vi "File Page - Get Stop Trigger.vi"(7 "File Ctl Refs":T1, 8 "error in (no error)":errorcluster, 11 "Item Ref in":T11 format="%.0x") -> (0 "error out":errorcluster, 3 "Item Ref out":T11 format="%.0x")   [LabVIEW 2015, in "Waveform Data Logger System Explorer.lvlib"]
uses:
  Waveform Data Logger System Explorer.lvlib
  <vilib>/NI Veristand/Custom Device API/Custom Device Item Ref.ctl
  Types/File Ctl Refs.ctl
  Types/File - Spec Ctl Refs.ctl
  Types/File - Wfm Ctl Refs.ctl
  Types/File - Settings Ctl Refs.ctl
  Classes/Log File Specifications/Log File Specification/File Conflict Operation.ctl
  Types/File - Start Trig Ctl Refs.ctl
  Shared/Types/Start Trigger.ctl
  Shared/Types/Default Trigger.ctl
  Shared/Types/Digital Trigger.ctl
  Shared/Types/Analog Trigger.ctl
  Shared/Types/In Range Trigger.ctl
  Shared/Types/Value Change Trigger.ctl
  Shared/Types/Boolean Trigger.ctl
  Types/Single Node Browser Data.ctl
  <vilib>/NI Veristand/UI Controls/Single Node Browser/Single Node Browser Ref.ctl
  NationalInstruments.VeriStand.SystemStorageUI
  <vilib>/NI Veristand/UI Controls/Single Node Browser/Callback Type.ctl
  <vilib>/NI Veristand/UI Controls/Single Node Browser/Net Event Data.ctl
  <vilib>/NI Veristand/UI Controls/Single Node Browser/Net Event.ctl
  Types/File - Stop Trig Ctl Refs.ctl
  Shared/Types/Stop Trigger.ctl
  Types/File - Advanced Ctl Refs.ctl
  Types/Log Timestamps.ctl
  Shared/Types/Trigger Direction.ctl
  Shared/Globals/Property Strings.vi
  <vilib>/NI Veristand/Custom Device API/Get Item Property (U16).vi
  <vilib>/NI Veristand/Custom Device API/Get Item Property (Double).vi
  Shared/Waveform Data Logger Shared.lvlib
  <vilib>/NI Veristand/Custom Device API/Custom Device API.lvlib
  Classes/Log File Specifications/Log File Specification/Log File Specification.lvclass
  <vilib>/NI Veristand/UI Controls/Single Node Browser/NI_VS UI Single Node Browser.lvlib
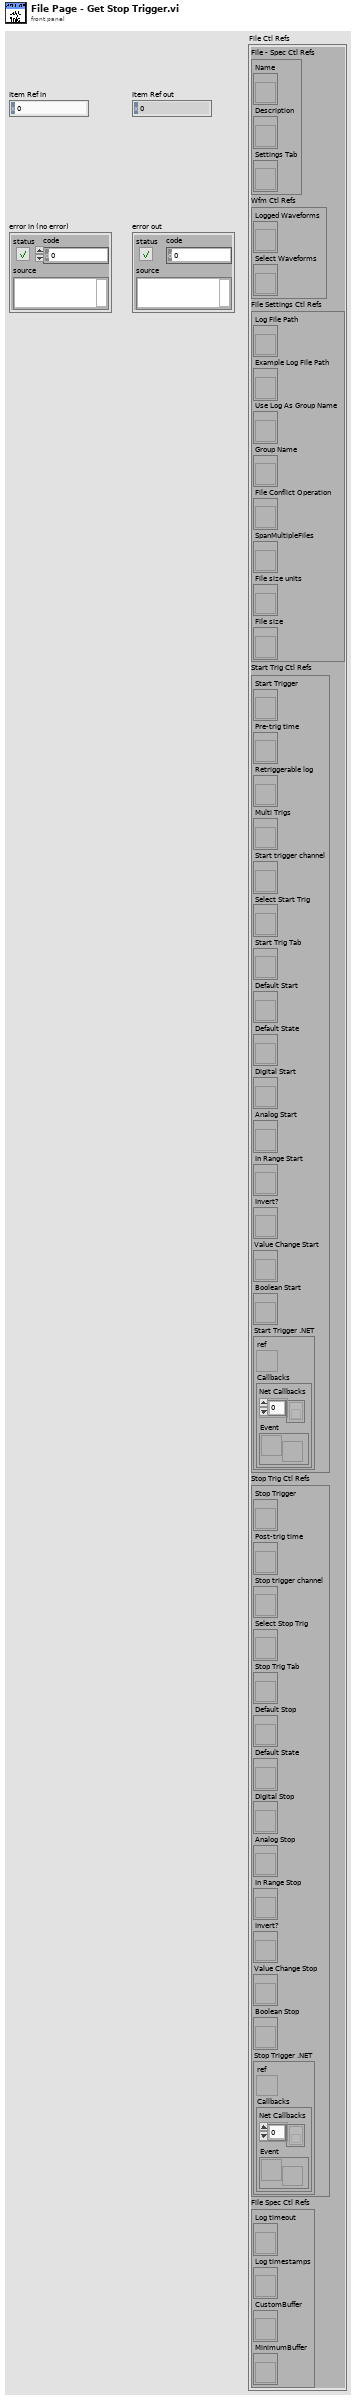
[diagram p1: front panel]
types:
  T1 = typedef "Waveform Data Logger System Explorer.lvlib/File Ctl Refs.ctl" = cluster{"File Spec Ctl Refs":T2, "Wfm Ctl Refs":T3, "File Settings Ctl Refs":T4, "Start Trig Ctl Refs":T5, "Stop Trig Ctl Refs":T9, "File Spec Ctl Refs":T10}
  T2 = typedef "Waveform Data Logger System Explorer.lvlib/File - Spec Ctl Refs.ctl" = cluster{"Name":refnum<vi>, "Description":refnum<vi>, "Settings Tab":refnum<vi>}
  T3 = typedef "Waveform Data Logger System Explorer.lvlib/File - Wfm Ctl Refs.ctl" = cluster{"Logged Waveforms":refnum<vi>, "Select Waveforms":refnum<vi>}
  T4 = typedef "Waveform Data Logger System Explorer.lvlib/File - Settings Ctl Refs.ctl" = cluster{"Log File Path":refnum<vi>, "Example Log File Path":refnum<vi>, "Use Log As Group Name":refnum<vi>, "Group Name":refnum<vi>, "File Conflict Operation":refnum<vi>, "SpanMultipleFiles":refnum<vi>, "File size units":refnum<vi>, "File size":refnum<vi>}
  T5 = typedef "Waveform Data Logger System Explorer.lvlib/File - Start Trig Ctl Refs.ctl" = cluster{"Start Trigger":refnum<vi>, "Pre-trig time":refnum<vi>, "Retriggerable log":refnum<vi>, "Multi Trigs":refnum<vi>, "Start trigger channel":refnum<vi>, "Select Start Trig":refnum<vi>, "Start Trig Tab":refnum<vi>, "Default Start":refnum<vi>, "Default State":refnum<vi>, "Digital Start":refnum<vi>, "Analog Start":refnum<vi>, "In Range Start":refnum<vi>, "Invert?":refnum<vi>, "Value Change Start":refnum<vi>, "Boolean Start":refnum<vi>, "Start Trigger .NET":T6}
  T6 = typedef "Waveform Data Logger System Explorer.lvlib/Single Node Browser Data.ctl" = cluster{"ref":T7, "Callbacks":T8}
  T7 = typedef "NI_VS UI Single Node Browser.lvlib/Single Node Browser Ref.ctl" = refnum<k24>
  T8 = typedef "NI_VS UI Single Node Browser.lvlib/Callback Type.ctl" = cluster{"Net Callbacks":refnum<k27>[], "Event":refnum<user-event>}
  T9 = typedef "Waveform Data Logger System Explorer.lvlib/File - Stop Trig Ctl Refs.ctl" = cluster{"Stop Trigger":refnum<vi>, "Post-trig time":refnum<vi>, "Stop trigger channel":refnum<vi>, "Select Stop Trig":refnum<vi>, "Stop Trig Tab":refnum<vi>, "Default Stop":refnum<vi>, "Default State":refnum<vi>, "Digital Stop":refnum<vi>, "Analog Stop":refnum<vi>, "In Range Stop":refnum<vi>, "Invert?":refnum<vi>, "Value Change Stop":refnum<vi>, "Boolean Stop":refnum<vi>, "Stop Trigger .NET":T6}
  T10 = typedef "Waveform Data Logger System Explorer.lvlib/File - Advanced Ctl Refs.ctl" = cluster{"Log timeout":refnum<vi>, "Log timestamps":refnum<vi>, "CustomBuffer":refnum<vi>, "MinimumBuffer":refnum<vi>}
  T11 = typedef "Custom Device API.lvlib/Custom Device Item Ref.ctl" = u64
  T12 = typedef "Waveform Data Logger Shared.lvlib/Trigger Direction.ctl" = enum16{"Start", "Stop"}
  T13 = typedef "Waveform Data Logger Shared.lvlib/Analog Trigger.ctl" = cluster{"Strict edge":bool, "Slope":enum16{"Rising", "Falling"}, "Threshold":dbl}
  T14 = typedef "Waveform Data Logger Shared.lvlib/Boolean Trigger.ctl" = cluster{"Value":dbl, "Operand":enum16{"Equal to", "Not equal to", "Less than", "Less than or equal", "Greater than", "Greater than or equal"}}
  T15 = typedef "Waveform Data Logger Shared.lvlib/Default Trigger.ctl" = cluster{"Default State":bool}
  T16 = typedef "Waveform Data Logger Shared.lvlib/Digital Trigger.ctl" = cluster{"Edge":enum16{"Rising", "Falling"}}
  T17 = typedef "Waveform Data Logger Shared.lvlib/In Range Trigger.ctl" = cluster{"High limit":dbl, "Low limit":dbl, "Invert?":bool}
  T18 = typedef "Waveform Data Logger Shared.lvlib/Value Change Trigger.ctl" = cluster{"Deadband":dbl}
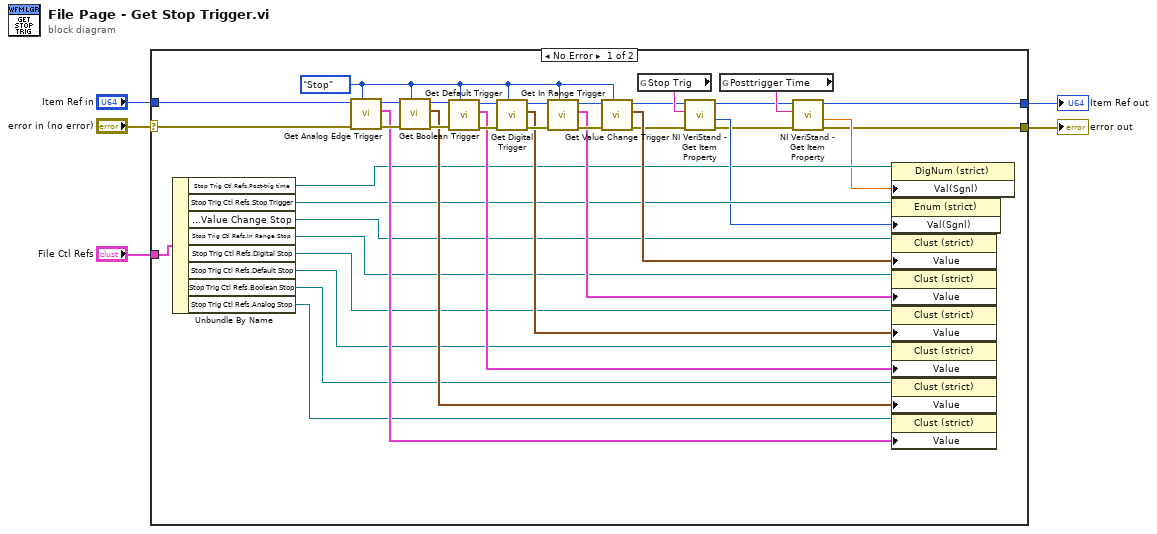
[diagram p0: block diagram]
diagram:
  n1 = case shown="No Error" "error in (no error)" {
    selector: "error in (no error)" -> [w25 w44]
    tunnel: [w7 w45] -> w5
    tunnel: [w6 w44] -> w4
    tunnel: "Item Ref in" -> [w26 w45]
    tunnel: "File Ctl Refs" -> [w24 _]
    frame No Error {
      w33 = Trigger_Direction."Stop" ("Trigger Direction")
      n2 = Unbundle By Name(w24) -> ("Stop Trig Ctl Refs.Post-trig time"=w9:refnum<vi>, "Stop Trig Ctl Refs.Stop Trigger"=w14:refnum<vi>, "Stop Trig Ctl Refs.Value Change Stop"=w18:refnum<vi>, "Stop Trig Ctl Refs.In Range Stop"=w19:refnum<vi>, "Stop Trig Ctl Refs.Digital Stop"=w20:refnum<vi>, "Stop Trig Ctl Refs.Default Stop"=w21:refnum<vi>, "Stop Trig Ctl Refs.Boolean Stop"=w22:refnum<vi>, "Stop Trig Ctl Refs.Analog Stop"=w23:refnum<vi>)
      n3 = call "Get Analog Edge Trigger.vi"("Trigger Direction"=w33, "error in (no error)"=w25, "Item Ref in"=w26) -> ("error out"=w42:errorcluster, "Analog Trigger"=w32:T13, "Item Ref out"=w43:T11)  [unwired: 6 in]
      n4 = call "Get Boolean Trigger.vi"("Trigger Direction"=w33, "error in (no error)"=w42, "Item Ref in"=w43) -> ("error out"=w40:errorcluster, "Boolean Trigger"=w31:T14, "Item Ref out"=w41:T11)  [unwired: 6 in]
      n5 = call "Get Default Trigger.vi"("Trigger Direction"=w33, "error in (no error)"=w40, "Item Ref in"=w41) -> ("error out"=w38:errorcluster, "Default Trigger"=w30:T15, "Item Ref out"=w39:T11)  [unwired: 6 in]
      n6 = call "Get Digital Trigger.vi"("Trigger Direction"=w33, "error in (no error)"=w38, "Item Ref in"=w39) -> ("error out"=w36:errorcluster, "Digital Trigger"=w29:T16, "Item Ref out"=w37:T11)  [unwired: 6 in]
      n7 = call "Get In Range Trigger.vi"("Trigger Direction"=w33, "error in (no error)"=w36, "Item Ref in"=w37) -> ("error out"=w34:errorcluster, "In Range Trigger"=w28:T17, "Item Ref out"=w35:T11)  [unwired: 6 in]
      n8 = call "Get Value Change Trigger.vi"("Trigger Direction"=w33, "error in (no error)"=w34, "Item Ref in"=w35) -> ("error out"=w15:errorcluster, "Value Change Trigger"=w27:T18, "Item Ref out"=w16:T11)  [unwired: 6 in]
      n9 = global read "Property Strings.vi" "Stop Trig"() -> (w17:string)
      n10 = call-poly <vilib>:"NI VeriStand - Get Item Property.vi"("error in (no error)"=w15, "Property Name"=w17, "Item Ref in"=w16) -> ("error out"=w10:errorcluster, "Value"=w13:u16, "Item Ref out"=w11:T11)  [unwired: 1 in, 5 out]
      n11 = global read "Property Strings.vi" "Posttrigger Time"() -> (w12:string)
      n12 = call-poly <vilib>:"NI VeriStand - Get Item Property.vi"("error in (no error)"=w10, "Property Name"=w12, "Item Ref in"=w11) -> ("error out"=w6:errorcluster, "Value"=w8:dbl, "Item Ref out"=w7:T11)  [unwired: 1 in, 5 out]
      n13 = property on="Property Node" class="DigNum (strict)"(reference=w9, "Val(Sgnl)"=w8) -> ()  [unwired: 1 in, 2 out]
      n14 = property on="Property Node" class="Enum (strict)"(reference=w14, "Val(Sgnl)"=w13) -> ()  [unwired: 1 in, 2 out]
      n15 = property class="Clust (strict)"(reference=w18, "Value"=w27) -> ()  [unwired: 1 in, 2 out]
      n16 = property class="Clust (strict)"(reference=w19, "Value"=w28) -> ()  [unwired: 1 in, 2 out]
      n17 = property class="Clust (strict)"(reference=w20, "Value"=w29) -> ()  [unwired: 1 in, 2 out]
      n18 = property class="Clust (strict)"(reference=w21, "Value"=w30) -> ()  [unwired: 1 in, 2 out]
      n19 = property class="Clust (strict)"(reference=w22, "Value"=w31) -> ()  [unwired: 1 in, 2 out]
      n20 = property class="Clust (strict)"(reference=w23, "Value"=w32) -> ()  [unwired: 1 in, 2 out]
    }
    frame Error {
    }
  }
  "error out" <- w4
  "Item Ref out" <- w5
